vi "LCD Display Example.vi"() -> ()   [LabVIEW 2016]
uses:
  <vilib>/Rock Robotics/SystemInterfaces/AI/FPGA_AIChannel.ctl
  <vilib>/Rock Robotics/SystemInterfaces/DIO/FPGA_DIOChannel.ctl
panel:
  in  "LCD Backlight":T1(ring)
  in  "DIO Channel":T2
  in  "Analog Channel":T3
  in  "stop":bool
  in  "Update Frequency":dbl(slide)=3.0 scale=1.0..20.0
  # "Set these controls before running the example"
  # "Change these controls while running the example"
  # "This example demonstrates how to write to an LCD connected to the Huskie Board.\n\nCurrently, the Huskie Board supports the Paralax Serial LCD (27976, 27977, 27979).\n\nThis example writes three lines to the LCD. If a 2 row LCD is used, only the last two lines will be visible. The information that is displayed on the first line is the battery voltage and if the robot is connected to the FMS. The information that is displayed on the second line is the voltage of the selected analog channel. The information that is displayed on the thbird line is the value of the selected DIO channel.\n\nThe update frequency control may be changed while the example is running to adjust how often the LCD is updated."
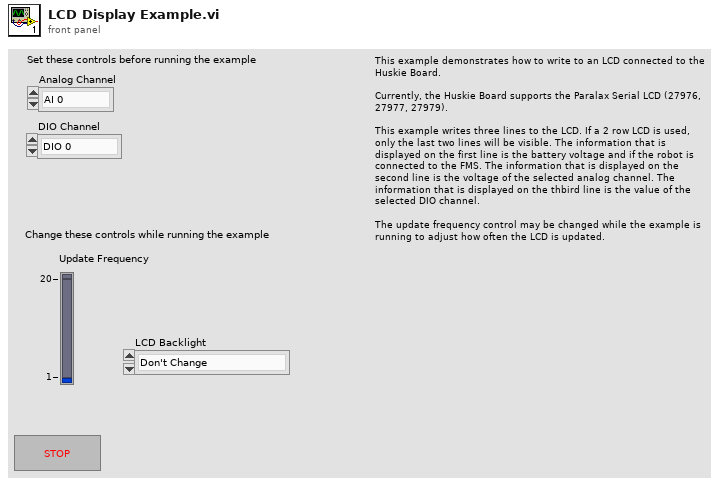
[diagram p1: front panel]
types:
  T1 = enum8{"Don't Change", "Backlight On", "Backlight Off"}
  T2 = typedef "FPGA_DIOChannel.ctl" = enum8{"DIO 0", "DIO 1", "DIO 2", "DIO 3", "DIO 4", "DIO 5", "DIO 6", "DIO 7", "DIO 8", "DIO 9", "DIO MXP 0", "DIO MXP 1", "DIO MXP 2", "DIO MXP 3", "DIO MXP 4", "DIO MXP 5", "DIO MXP 6", "DIO MXP 7", "DIO MXP 8", "DIO MXP 9", "DIO MXP 10", "DIO MXP 11", "DIO MXP 12", "DIO MXP 13", "DIO MXP 14", "DIO MXP 15", "SPI Port CS1", "SPI Port CS2", "SPI Port CS3", "SPI Port MISO", "SPI Port MOSI", "Invalid"}
  T3 = typedef "FPGA_AIChannel.ctl" = enum8{"AI 0", "AI 1", "AI 2", "AI 3", "AI MXP 0", "AI MXP 1", "AI MXP 2", "AI MXP 3", "Invalid"}
  T4 = typedef "WPI_SerialPortRef.ctl" = cluster{"DevStatus":errorcluster, "Serial Port Name":refnum<visa-resource-name>}
  T5 = typedef "WPI_AnalogChannelDevRef.ctl" = cluster{"DevStatus":errorcluster, "Analog Channel":T3}
  T6 = typedef "WPI_DigitalInputDevRef.ctl" = cluster{"DevStatus":errorcluster, "DIO Channel":T2}
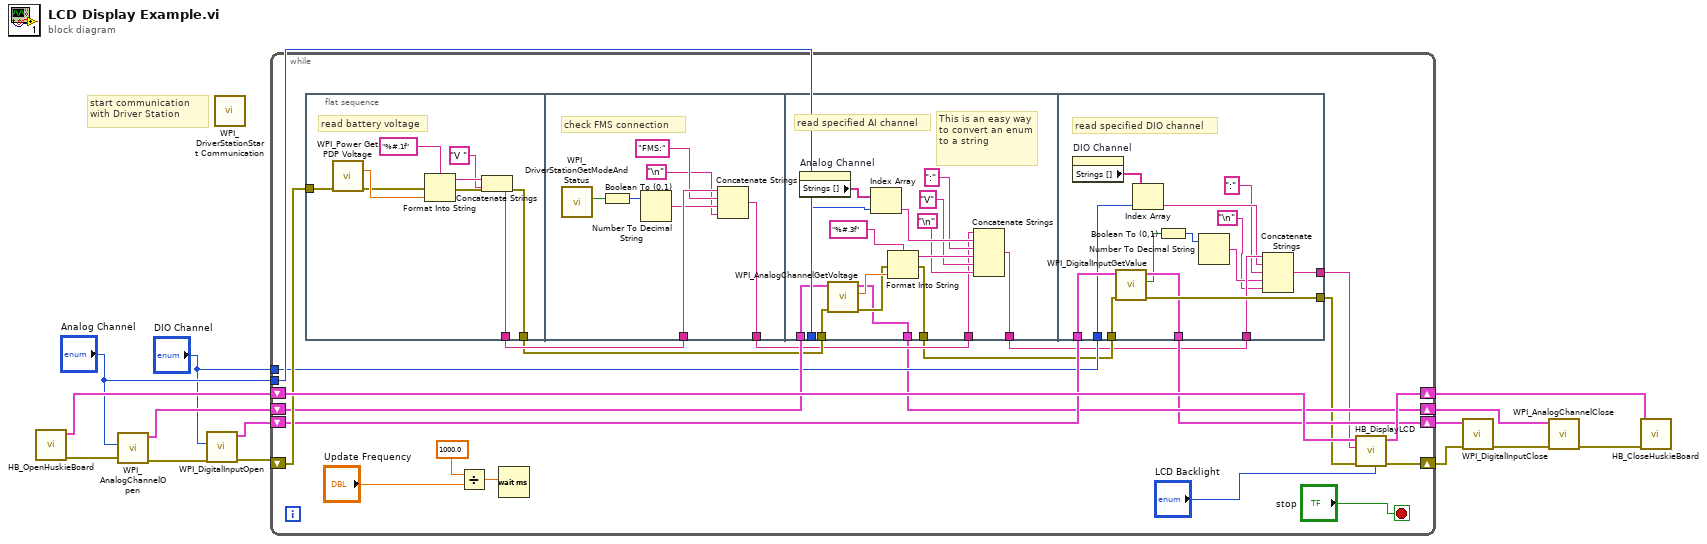
[diagram p0: block diagram]
diagram:
  # "start communication with Driver Station"
  n1 = call <vilib>:"HB_OpenHuskieBoard.vi"() -> ("error out"=w12:errorcluster, "HBDeviceRef"=w14:T4)  [unwired: 10 in]
  n2 = call <vilib>:"WPI_AnalogChannelOpen.vi"("error in (no error)"=w12, "Analog Channel"="Analog Channel") -> ("error out"=w11:errorcluster, "AIDeviceRef"=w9:T5)  [unwired: 8 in]
  n3 = call <vilib>:"WPI_DigitalInputOpen.vi"("error in (no error)"=w11, "DIO Channel"="DIO Channel") -> ("error out"=w10:errorcluster, "DigitalInputDevRef"=w8:T6)  [unwired: 8 in]
  n4 = call <vilib>:"WPI_DriverStationStart Communication.vi"() -> ()  [unwired: 2 in, 10 out]
  n5 = while {
    shift-right: [w31] -> w13
    shift-left: w14 -> [w32]
    shift-right: [w30] -> w6
    shift-left: w10 -> [w29]
    tunnel: "Analog Channel" -> [w25]
    shift-right: [w20] -> w3
    shift-left: w9 -> [w27]
    shift-right: [w19] -> w2
    shift-left: w8 -> [w23]
    tunnel: "DIO Channel" -> [w22]
    stop <- "stop" stop-if-true
    n6 = flat-sequence {
      tunnel: w29 -> [w43]
      tunnel: [w38] -> w26
      tunnel: [w37] -> w28
      tunnel: w28 -> [w49]
      tunnel: [w45] -> w24
      tunnel: w27 -> [w66]
      tunnel: w26 -> [w65]
      tunnel: w25 -> [w62]
      tunnel: [w56] -> w18
      tunnel: w24 -> [w55]
      tunnel: [w54] -> w21
      tunnel: [w53] -> w20
      tunnel: w23 -> [w79]
      tunnel: w22 -> [w78]
      tunnel: w21 -> [w77]
      tunnel: [w76] -> w16
      tunnel: [w75] -> w19
      tunnel: w18 -> [w73]
      tunnel: [w68] -> w17
      frame #0 {
        # "read battery voltage"
        n7 = call <vilib>:"WPI_Power Get PDP Voltage.vi"("error in"=w43) -> ("voltage (V)"=w42:dbl, "error out"=w41:errorcluster)  [unwired: 13 in]
        n8 = Format Into String(format string="%#.1f", error in=w41, w42) -> (resulting string=w40:string, error out=w38:errorcluster)  [unwired: 1 in]
        n9 = Concatenate Strings(w40, "V " ("string")) -> (w37:string)
      }
      frame #1 {
        # "check FMS connection"
        n10 = call <vilib>:"WPI_DriverStationGetModeAndStatus.vi"() -> ("FMS Attached"=w51:bool)  [unwired: 10 in, 1 out]
        n11 = Boolean To (0,1)(Boolean=w51) -> (0, 1=w50:i16)
        n12 = Number To Decimal String(number=w50) -> (decimal integer string=w47:string)  [unwired: 1 in]
        n13 = Concatenate Strings(w49, "FMS:" ("string"), w47, "\n") -> (w45:string)
      }
      frame #2 {
        # "This is an easy way to convert an enum to a string"
        # "read specified AI channel"
        n14 = property on="Analog Channel" class="Enum (strict)"() -> ("Strings []"=w67:string[])  [unwired: 2 in, 2 out]
        n15 = call <vilib>:"WPI_AnalogChannelGetVoltage.vi"("error in (no error)"=w65, "AIDeviceRef"=w66) -> ("error out"=w63:errorcluster, "Voltage"=w64:dbl, "AIDeviceRef"=w53:T5)  [unwired: 7 in]
        n16 = Index Array(array=w67, index=w62) -> (element=w61:string)
        n17 = Format Into String(format string="%#.3f", error in=w63, w64) -> (resulting string=w59:string, error out=w54:errorcluster)  [unwired: 1 in]
        n18 = Concatenate Strings(w55, w61, ":" ("string"), w59, "V" ("string"), "\n") -> (w56:string)
      }
      frame #3 {
        # "read specified DIO channel"
        n19 = property on="DIO Channel" class="Enum (strict)"() -> ("Strings []"=w81:string[])  [unwired: 2 in, 2 out]
        n20 = call <vilib>:"WPI_DigitalInputGetValue.vi"("error in (no error)"=w77, "DigitalInputDevRef"=w79) -> ("error out"=w76:errorcluster, "Value"=w74:bool, "DigitalInputDevRef"=w75:T6)  [unwired: 7 in]
        n21 = Index Array(array=w81, index=w78) -> (element=w72:string)
        n22 = Boolean To (0,1)(Boolean=w74) -> (0, 1=w80:i16)
        n23 = Number To Decimal String(number=w80) -> (decimal integer string=w70:string)  [unwired: 1 in]
        n24 = Concatenate Strings(w73, w72, ":" ("string"), w70, "\n") -> (w68:string)
      }
    }
    n25 = Divide(x=1000.0, y="Update Frequency") -> (x/y=w35:dbl)
    n26 = Wait (ms)(milliseconds to wait=w35) -> ()  [unwired: 1 out]
    n27 = call <vilib>:"HB_DisplayLCD.vi"("LCD Backlight"="LCD Backlight", "error in (no error)"=w16, "Display String"=w17, "HBDeviceRef"=w32) -> ("error out"=w30:errorcluster, "HBDeviceRef"=w31:T4)  [unwired: 6 in]
  }
  n28 = call <vilib>:"WPI_DigitalInputClose.vi"("error in (no error)"=w6, "DigitalInputDevRef"=w2) -> ("error out"=w5:errorcluster)  [unwired: 9 in]
  n29 = call <vilib>:"WPI_AnalogChannelClose.vi"("error in (no error)"=w5, "AIDeviceRef"=w3) -> ("error out"=w4:errorcluster)  [unwired: 9 in]
  n30 = call <vilib>:"HB_CloseHuskieBoard.vi"("error in (no error)"=w4, "HBDeviceRef"=w13) -> ()  [unwired: 9 in, 1 out]
